vi "Scale Updated.vi"(8 "error in":errorcluster, 10 "Scale Max":i32) -> (0 "error out":errorcluster)   [LabVIEW 2019, in "Panther Dashboard.lvlib"]
doc: "_____\nCreated using DQMH Event Scripter 6.1.0.128."
uses:
  Panther Dashboard.lvlib
  Scale Updated Argument--cluster.ctl
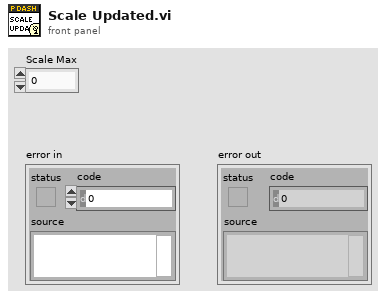
[diagram p1: front panel]
types:
  T1 = typedef "Panther Dashboard.lvlib/Scale Updated Argument--cluster.ctl" = cluster{"Scale Max":i32}
  T2 = typedef "Panther Dashboard.lvlib/Broadcast Events--cluster.ctl" = cluster{"Module Did Init":refnum<user-event>, "Status Updated":refnum<user-event>, "Error Reported":refnum<user-event>, "Module Did Stop":refnum<user-event>, "Update Module Execution Status":refnum<user-event>, "References Updated":refnum<user-event>, "Projects Updated":refnum<user-event>, "Targets Updated":refnum<user-event>, "Progress updated":refnum<user-event>, "Scale Updated":refnum<user-event>}
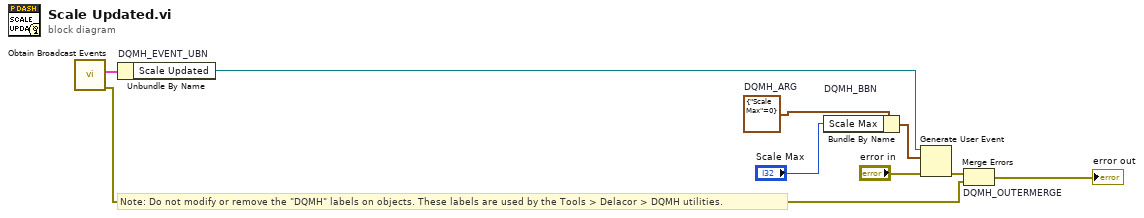
[diagram p0: block diagram]
diagram:
  w4 = T1 {"Scale Max"=0}  # DQMH_ARG
  # "Note: Do not modify or remove the \"DQMH\" labels on objects. These labels are used by the Tools > Delacor > DQMH utilities."
  n1 = call "Obtain Broadcast Events.vi"() -> ("error out"=w2:errorcluster, "Panther Dashboard Broadcast Events"=w1:T2)  [unwired: 10 in]
  n2 = Unbundle By Name "DQMH_EVENT_UBN"(w1) -> ("Scale Updated"=w6:refnum<user-event>)
  n3 = Bundle By Name "DQMH_BBN"(cluster=w4, "Scale Max"="Scale Max") -> (w7:T1)
  n4 = Generate User Event(user event=w6, event data cluster=w7, error in="error in") -> (error out=w5:errorcluster)  [unwired: 1 in, 1 out]
  n5 = Merge Errors "DQMH_OUTERMERGE"(w5, w2) -> (→"error out":errorcluster)
